vi "upload.start_part_upload.vi"(6 "Part Number":i32, 8 "error in":errorcluster, 9 "timeout (ms)":i32=300000, 10 "File Part Binary":string, 11 "Multipart Upload":refnum<class "Multipart Upload.lvclass">) -> (0 "error out":errorcluster, 3 "Multipart Upload out":refnum<class "Multipart Upload.lvclass">)   [LabVIEW 2020, in "Multipart Upload.lvclass"]
uses:
  Multipart Upload.lvclass
  Multipart Upload.lvclass/Multipart Upload.ctl
  upload.part_core.vi
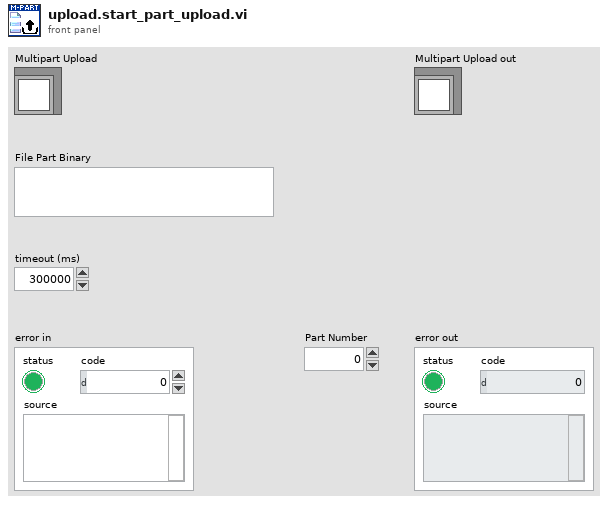
[diagram p1: front panel]
types:
  T1 = map{i32, cluster{"url":string, "headers":map{string, string}}}
  T2 = cluster{"url":string, "headers":map{string, string}}
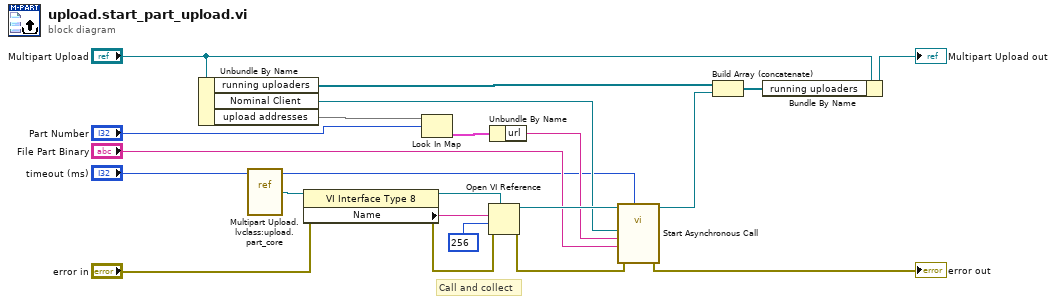
[diagram p0: block diagram]
diagram:
  # "Call and collect"
  n1 = Unbundle By Name("Multipart Upload") -> ("running uploaders"=w11:refnum<vi>[], "Nominal Client"=w3:refnum<class "Nominal Client.lvclass">, "upload addresses"=w7:T1)
  n2 = vi-ref "Multipart Upload.lvclass:upload.part_core.vi"() -> (w17:refnum<vi>)
  n3 = property class="VI Interface Type 8"(reference=w17, error in="error in") -> (reference out=w15:refnum<vi>, error out=w13:errorcluster, "Name"=w16:string)
  n4 = Look In Map(map=w7, key="Part Number") -> (value=w5:T2)  [unwired: 1 in, 1 out]
  n5 = Open VI Reference(type specifier VI Refnum (for type only)=w15, vi path=w16, options=256, error in (no error)=w13) -> (vi reference=w20:refnum<vi>, error out=w19:errorcluster)  [unwired: 2 in]
  n6 = Unbundle By Name(w5) -> ("url"=w4:string)
  n7 = call-by-ref "Start Asynchronous Call"(reference=w20, error in=w19, "timeout (ms)"="timeout (ms)", "Body"="File Part Binary", "Full Path"=w4, "Nominal Client"=w3) -> (reference out=w10:refnum<vi>, error out=→"error out":errorcluster)  [unwired: 6 in, 2 out]
  n8 = Build Array (concatenate)(w11, w10) -> (w2:refnum<vi>[])
  n9 = Bundle By Name(cluster="Multipart Upload", "running uploaders"=w2) -> (→"Multipart Upload out":refnum<class "Multipart Upload.lvclass">)
